vi "dataScopes.set.vi"(8 "error in":errorcluster, 10 "datascopes":T1, 11 "asset in":refnum<class "asset.lvclass">) -> (0 "error out":errorcluster, 3 "asset out":refnum<class "asset.lvclass">)   [LabVIEW 2020, in "asset.lvclass"]
uses:
  asset.lvclass
  nominal types/dataScope/data_scopes.ctl
  nominal types/dataScope/data_scope.ctl
  nominal types/dataScope/data_source.ctl
  nominal types/dataScope/type.ctl
  nominal types/dataScope/offset.ctl
  asset.lvclass/asset.ctl
  Nominal Client/Nominal Client.lvclass/Nominal Client.ctl
  Nominal Client/error.vi
  Nominal Client/trace.payload_sent.vi
  Nominal Client/trace.payload_received.vi
  Nominal Client/create.authorization_header.vi
  Nominal Client/error.vi/859f8e04-e495-489b-b5b4-7ac163f56130.vi
  Nominal Client/trace.calling_method.vi
  <vilib>/JDP Science/JDP Science Common Utilities/Trim Whitespace__JDP.vi
  <vilib>/AdvancedString/1D String Array to Delimited String.vi
  Nominal Client/api_token.get.vi
  <vilib>/Utility/libraryn.llb/Get File Extension.vi
  Nominal Client/log_file.write.vi
  <vilib>/JDP Science/JSONtext/Get all Object Items.vi
  <vilib>/Utility/error.llb/Error Cluster From Error Code.vi
  <vilib>/JDP Science/JSONtext/JSON text to Variant.vi
  <vilib>/JDP Science/JSONtext/LVClass Serializer/JSONtext LVClass Serializer.lvclass
  <vilib>/addons/_JKI.lib/REST Client/classes/Response Headers/Response Headers.lvclass
  <vilib>/addons/_JKI.lib/REST Client/classes/REST Client/REST Client.lvclass
  Nominal Client/Nominal Client.lvclass
  nominal types/dataScope/dataScopes.lvlib
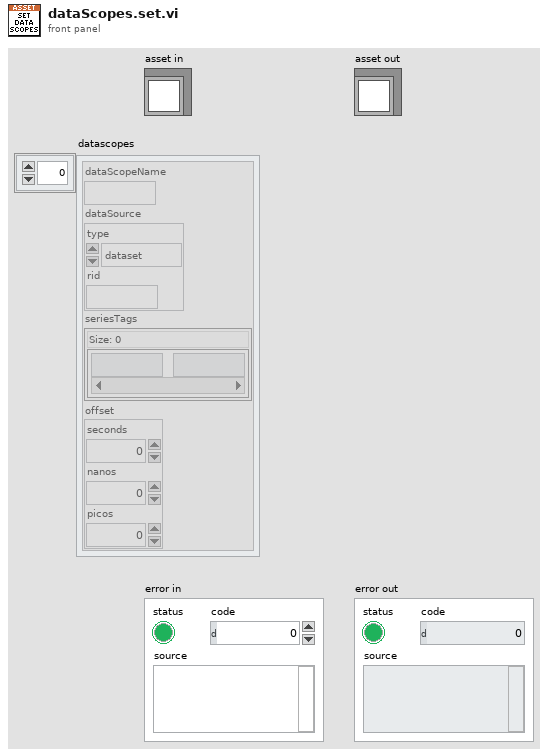
[diagram p1: front panel]
types:
  T1 = typedef "dataScopes.lvlib/data_scopes.ctl" = T2[]
  T2 = typedef "dataScopes.lvlib/data_scope.ctl" = cluster{"dataScopeName":string, "dataSource":T3, "seriesTags":map{string, string}, "offset":T5}
  T3 = typedef "dataScopes.lvlib/data_source.ctl" = cluster{"type":T4, "rid":string}
  T4 = typedef "dataScopes.lvlib/type.ctl" = enum16{"dataset", "connection", "logSet", "video"}
  T5 = typedef "dataScopes.lvlib/offset.ctl" = cluster{"seconds":i32, "nanos":i32, "picos":i32}
  T6 = typedef "dataScopes.lvlib/links.ctl" = cluster{"URL":string, "Title":string}[]
  T7 = cluster{"rid":string, "title":string, "properties":refnum<class "properties.lvclass">, "labels":refnum<class "labels.lvclass">, "Links":T6, "datascopes":T1, "createdAt":timestamp, "updatedAt":timestamp, "attachments":refnum<class "labels.lvclass">, "isStaged":bool, "isArchived":bool, "description":string, "createdBy":string, "type":string}
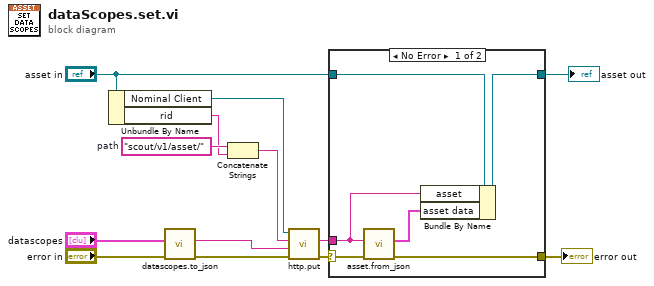
[diagram p0: block diagram]
diagram:
  w12 = "scout/v1/asset/"  # path
  n1 = Unbundle By Name("asset in") -> ("Nominal Client"=w13:refnum<class "Nominal Client.lvclass">, "rid"=w10:string)
  n2 = call "datascopes.to_json.vi"("error in"="error in", "datascopes"="datascopes") -> ("error out"=w2:errorcluster, "json"=w3:string)  [unwired: 8 in]
  n3 = Concatenate Strings(w12, w10) -> (w11:string)
  n4 = call "http.put.vi"("error in"=w2, "Body"=w3, "Path"=w11, "Nominal Client in"=w13) -> ("error out"=w9:errorcluster, "Response"=w6:string)  [unwired: 4 in, 2 out]
  n5 = case shown="No Error" w9 {
    selector: w9 -> [w19 w21]
    tunnel: [w18 w21] -> w8
    tunnel: "asset in" -> [w17 w20]
    tunnel: w6 -> [w15 _]
    tunnel: [w14 w20] -> w5
    frame No Error {
      n6 = call "asset.from_json.vi"("error in"=w19, "asset"=w15) -> ("error out"=w18:errorcluster, "Asset Data"=w16:T7)  [unwired: 8 in]
      n7 = Bundle By Name(cluster=w17, "asset"=w15, "asset data"=w16) -> (w14:refnum<class "asset.lvclass">)
    }
    frame Error {
    }
  }
  "asset out" <- w5
  "error out" <- w8
